vi "Check Data.vi"(10 "Display State":T2 caption="State", 11 "Data In":T1) -> (2 "Changed":bool, 3 "Data Out":T1)   [LabVIEW 2020, in "PXISlotGP.xctl"]
uses:
  PXISlotGP.xctl
  State.ctl
  PXISlot XControl/Connector Type.ctl
  AOAIRefs.ctl
  Data.ctl
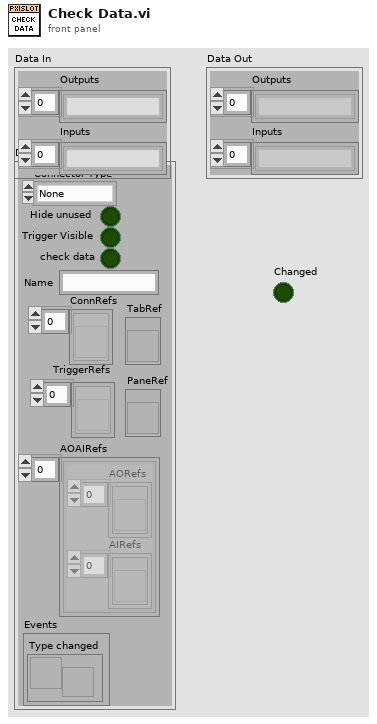
[diagram p1: front panel]
types:
  T1 = typedef "PXISlotGP.xctl/Data.ctl" = cluster{"Outputs":string[], "Inputs":string[]}
  T2 = typedef "PXISlotGP.xctl/State.ctl" = cluster{"Connector Type":T3, "Hide unused":bool, "Trigger Visible":bool, "TabRef":refnum<vi>, "ConnRefs":refnum<vi>[], "PaneRef":refnum<vi>, "AOAIRefs":T4[], "TriggerRefs":refnum<vi>[], "check data":bool, "Name":string, "Events":cluster{"Type changed":refnum<user-event>}}
  T3 = typedef "Connector Type.ctl" = enum16{"None", "PXI-4461", "BNC-2110", "BNC-2090", "PXIe-4463", "PXIe-4464"}
  T4 = typedef "AOAIRefs.ctl" = cluster{"AORefs":refnum<vi>[], "AIRefs":refnum<vi>[]}
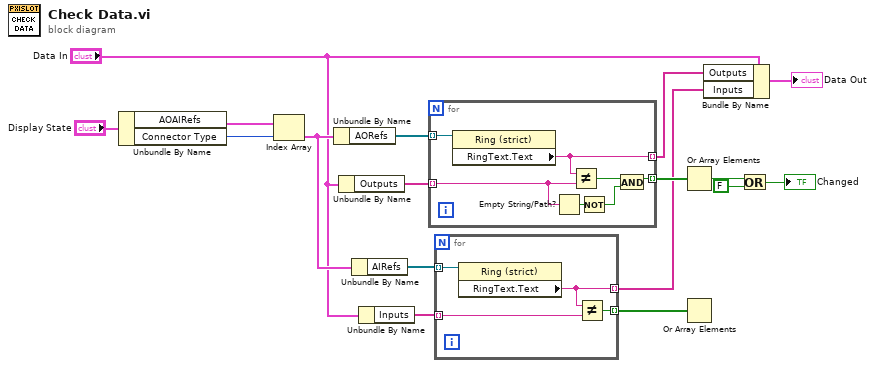
[diagram p0: block diagram]
diagram:
  n1 = Unbundle By Name("Display State") -> ("AOAIRefs"=w16:T4[], "Connector Type"=w15:T3)
  n2 = Index Array(array=w16, index=w15) -> (element=w12:T4)
  n3 = Unbundle By Name(w12) -> ("AORefs"=w14:refnum<vi>[])
  n4 = Unbundle By Name("Data In") -> ("Outputs"=w13:string[])
  n5 = Unbundle By Name(w12) -> ("AIRefs"=w11:refnum<vi>[])
  n6 = Unbundle By Name("Data In") -> ("Inputs"=w9:string[])
  n7 = for {
    tunnel: w14 -> [w24] mode=indexing
    tunnel: [w23] -> w3 mode=indexing
    tunnel: w13 -> [w20] mode=indexing
    tunnel: [w21] -> w8 mode=indexing
    n8 = property class="Ring (strict)"(reference=w24) -> ("RingText.Text"=w23:string)  [unwired: 1 in, 2 out]
    n9 = Empty String/Path?(string/path=w20) -> (empty?=w19:bool)
    n10 = Not Equal?(x=w23, y=w20) -> (x != y?=w22:bool)
    n11 = Not(x=w19) -> (.not. x?=w18:bool)
    n12 = And(x=w22, y=w18) -> (x .and. y?=w21:bool)
  }
  n13 = for {
    tunnel: w11 -> [w28] mode=indexing
    tunnel: [w27] -> w2 mode=indexing
    tunnel: w9 -> [w26] mode=indexing
    tunnel: [w25] -> w7 mode=indexing
    n14 = property class="Ring (strict)"(reference=w28) -> ("RingText.Text"=w27:string)  [unwired: 1 in, 2 out]
    n15 = Not Equal?(x=w27, y=w26) -> (x != y?=w25:bool)
  }
  n16 = Or Array Elements(Boolean array=w8) -> (logical OR=w6:bool)
  n17 = Or Array Elements(Boolean array=w7) -> ()  [unwired: 1 out]
  n18 = Bundle By Name(cluster="Data In", "Outputs"=w3, "Inputs"=w2) -> (→"Data Out":T1)
  n19 = Or(x=w6, y=FALSE) -> (x .or. y?=→"Changed":bool)
